vi "Is OD Entry.vi"(8 "error in":errorcluster, 11 "Section Name in":refnum<class "Section Name.lvclass">) -> (0 "error out":errorcluster, 1 "Is OD Entry?":bool, 2 "Index":u16 format="%.0x", 3 "Section Name out":refnum<class "Section Name.lvclass">, 4 "Is Sub-Entry?":bool)   [LabVIEW 2024, in "Electronic Datasheet.lvlib" / "Section Name.lvclass"]
uses:
  Section Name.lvclass
  Section Name.lvclass/Section Name.ctl
  <vilib>/regexp/Match Regular Expression.xnode
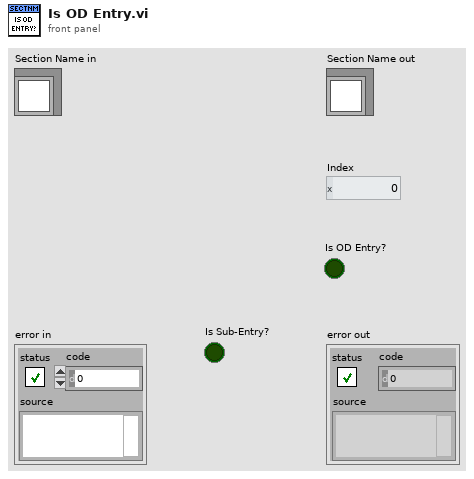
[diagram p1: front panel]
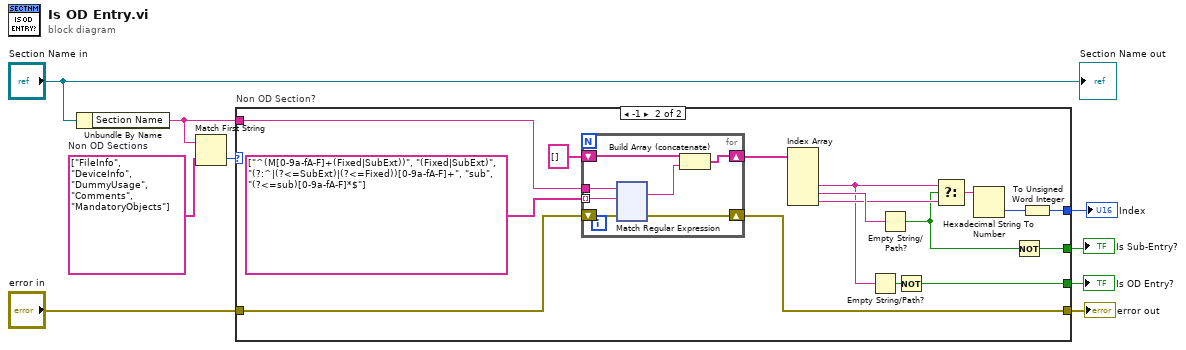
[diagram p0: block diagram]
diagram:
  w4 = string[] ["FileInfo", "DeviceInfo", "DummyUsage", "Comments", "MandatoryObjects"]  # Non OD Sections
  n1 = Unbundle By Name("Section Name in") -> ("Section Name"=w2:string)
  n2 = Match First String(2:w4, 3:w2) -> (0:w3:i32)  [unwired: 1 out]
  n3 = case "Non OD Section?" shown="-1" w3 {
    tunnel: [_ w23] -> w9
    tunnel: [_ w14] -> w8
    tunnel: "error in" -> [w10 w20]
    tunnel: [w10 w19] -> w6
    tunnel: w2 -> [_ w18]
    tunnel: [_ w12] -> w1
    frame Default {
    }
    frame -1 {
      n4 = for {
        tunnel: string[] ["^(M[0-9a-fA-F]+(Fixed|SubExt))", "(Fixed|SubExt)", "(?:^|(?<=SubExt)|(?<=Fixed))[0-9a-fA-F]+", "sub", "(?<=sub)[0-9a-fA-F]*$"] -> [w33] mode=indexing
        shift-right: [w31] -> w24
        shift-left: string[] [] -> [w32]
        tunnel: w18 -> [w29]
        shift-right: [w27] -> w19
        shift-left: w20 -> [w28]
        n5 = xnode "Match Regular Expression"("input string"=w29, "regular expression"=w33, "error in"=w28) -> ("whole match"=w30:string, "error out"=w27:errorcluster)  [unwired: 3 in, 3 out]
        n6 = Build Array (concatenate)(w32, w30) -> (w31:string[])
      }
      n7 = Index Array(array=w24) -> (element #3=w15:string, element #4=w22:string, element #5=w16:string)  [unwired: 5 in, 2 out]
      n8 = Empty String/Path?(string/path=w15) -> (empty?=w21:bool)
      n9 = Empty String/Path?(string/path=w22) -> (empty?=w13:bool)
      n10 = Not(x=w21) -> (.not. x?=w14:bool)
      n11 = Select(t=w15, s=w13, f=w16) -> (s? t:f=w17:string)
      n12 = Hexadecimal String To Number(string=w17) -> (number=w26:u32)  [unwired: 2 in, 1 out]
      n13 = Not(x=w13) -> (.not. x?=w12:bool)
      n14 = To Unsigned Word Integer(number=w26) -> (unsigned 16bit integer=w23:u16)
    }
  }
  "error out" <- w6
  "Index" <- w9
  "Is OD Entry?" <- w8
  "Is Sub-Entry?" <- w1
  "Section Name out" <- "Section Name in"
